vi "Theme5_Topic1_qn22.vi"(9 "RefPrevious":refnum<vi>, 10 "RefNext":refnum<vi>, 11 "connection reference":T1) -> (2 "AnsIndicator":refnum<vi>[](array[refnum]))   [LabVIEW 2013]
uses:
  why.vi
  Precontrol.vi
  <vilib>/addons/database/Connection.llb/Conn ObjectReference.ctl
  <vilib>/addons/database/NI_Database_API.lvlib
panel:
  out "Why?":string
  out "DInd":bool
  out "CInd":bool
  out "BInd":bool
  out "AInd":bool
  in  "ABCD":enum32{"No Selection", "A", "B", "C", "D"}(radio)
  out "MCQ_Randomized":string[](array[string])
  # "How can you we make or create static electricity?"
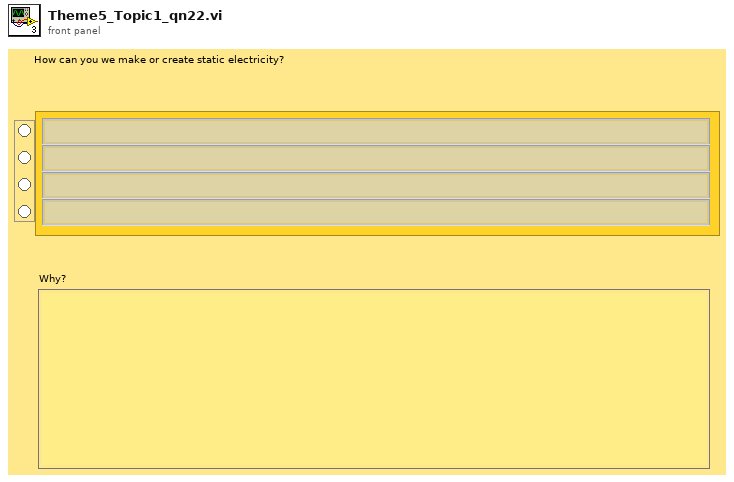
[diagram p1: front panel]
types:
  T1 = typedef "NI_Database_API.lvlib/Conn ObjectReference.ctl" = refnum<k1>
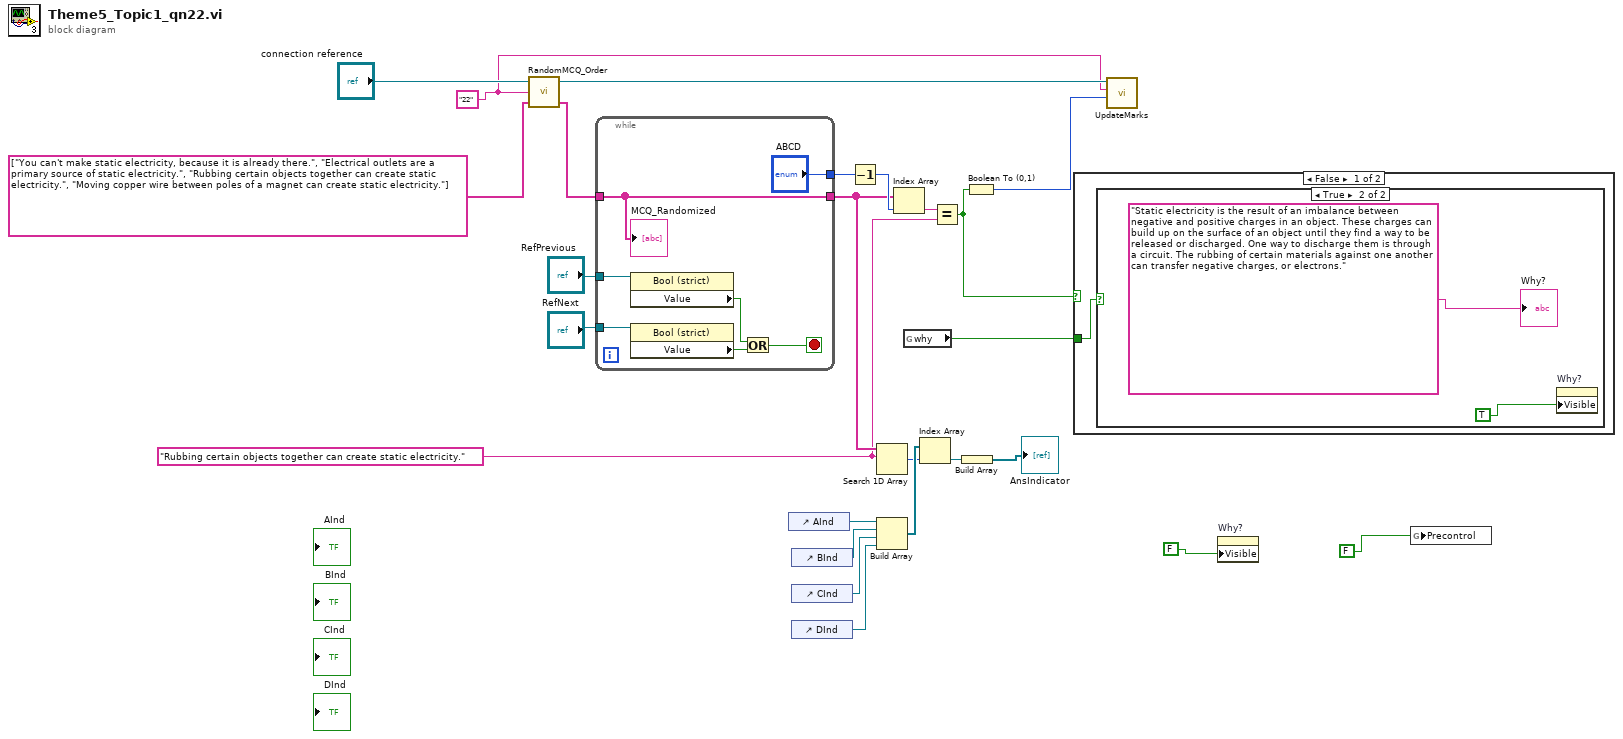
[diagram p0: block diagram]
diagram:
  w11 = "Rubbing certain objects together can create static electricity." ("element")
  w3 = "22" ("Questions_Ordered")
  n1 = call "RandomMCQ_Order.vi"("MCQ_Ordered"=string[] ["You can't make static electricity, because it is already there.", "Electrical outlets are a primary source of static electricity.", "Rubbing certain objects together can create static electricity.", "Moving copper wire between poles of a magnet can create static electricity."], "Questions_Ordered"=w3, "connection reference"="connection reference") -> ("MCQ_Randomized"=w25:string[], "connection reference out"=w9:T1)  [unwired: 1 in]
  n2 = while {
    tunnel: ["ABCD"] -> w15
    tunnel: w25 -> [w27]
    tunnel: [w27] -> w13
    tunnel: "RefNext" -> [w28]
    tunnel: "RefPrevious" -> [w29]
    stop <- w26 stop-if-true
    n3 = property class="Bool (strict)"(reference=w29) -> ("Value"=w31:bool)  [unwired: 1 in, 2 out]
    n4 = property class="Bool (strict)"(reference=w28) -> ("Value"=w30:bool)  [unwired: 1 in, 2 out]
    n5 = Or(x=w31, y=w30) -> (x .or. y?=w26:bool)
    "MCQ_Randomized" <- w27
  }
  n6 = control-ref of="AInd"() -> (w22:refnum<vi>)
  n7 = control-ref of="BInd"() -> (w21:refnum<vi>)
  n8 = control-ref of="CInd"() -> (w20:refnum<vi>)
  n9 = control-ref of="DInd"() -> (w19:refnum<vi>)
  n10 = Decrement(x=w15) -> (x-1=w14:enum32{"No Selection", "A", "B", "C", "D"})
  n11 = Search 1D Array(1D array=w13, element=w11) -> (index of element=w17:i32)  [unwired: 1 in]
  n12 = Build Array(w22, w21, w20, w19) -> (w18:refnum<vi>[])
  n13 = Index Array(array=w13, index=w14) -> (element=w12:string)
  n14 = global read "why.vi" "why"() -> (w2:bool)
  n15 = Index Array(array=w18, index=w17) -> (element=w16:refnum<vi>)
  n16 = Equal?(x=w12, y=w11) -> (x = y?=w5:bool)
  n17 = Build Array(w16) -> (→"AnsIndicator":refnum<vi>[])
  n18 = Boolean To (0,1)(Boolean=w5) -> (0, 1=w6:i16)
  n19 = case shown="False" w5 {
    tunnel: w2 -> [w33 _]
    frame False {
      n20 = case shown="True" w33 {
        frame False {
        }
        frame True {
          n21 = property on="Why?" class="Str"("Visible"=TRUE) -> ()  [unwired: 2 in, 2 out]
          "Why?" <- "Static electricity is the result of an imbalance between negative and positive charges in an object. These charges can build up on the surface of an object until they find a way to be released or discharged. One way to discharge them is through a circuit. The rubbing of certain materials against one another can transfer negative charges, or electrons."
        }
      }
    }
    frame True {
    }
  }
  n22 = call "UpdateMarks.vi"("MarksEarned"=w6, "QuestionsNo_Ordered"=w3, "connection reference"=w9) -> ()  [unwired: 9 in]
  n23 = property on="Why?" class="Str"("Visible"=FALSE) -> ()  [unwired: 2 in, 2 out]
  n24 = global write "Precontrol.vi" "Precontrol"(FALSE) -> ()
